vi "test Set Version on Close.vi"(8 "error in (no error)":errorcluster, 11 "TestCase in":refnum<class "Configuration Tests.lvclass">) -> (0 "error out":errorcluster, 3 "TestCase out":refnum<class "Configuration Tests.lvclass">)   [LabVIEW 2017, in "Configuration Tests.lvclass"]
uses:
  Configuration Tests.lvclass
  Typedefs/DSF Version Info.ctl
  <vilib>/addons/_JKI Toolkits/VI Tester/TestCase.llb/TestCase.lvclass
  Classes/Configuration/Configuration Session.lvclass
  DSF Core.lvlib
  C:/Program Files (x86)/National Instruments/LabVIEW 2017/vi.lib/addons/_JKI Toolkits/VI Tester/TestCase.llb/TestCase.lvclass
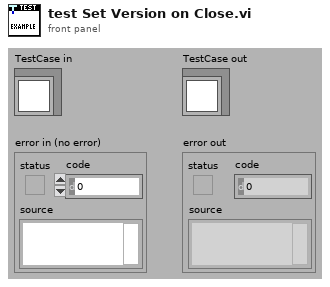
[diagram p1: front panel]
types:
  T1 = typedef "DSF Core.lvlib/DSF Version Info.ctl" = cluster{"major":u32, "minor":u32, "fix":u32, "build":string}
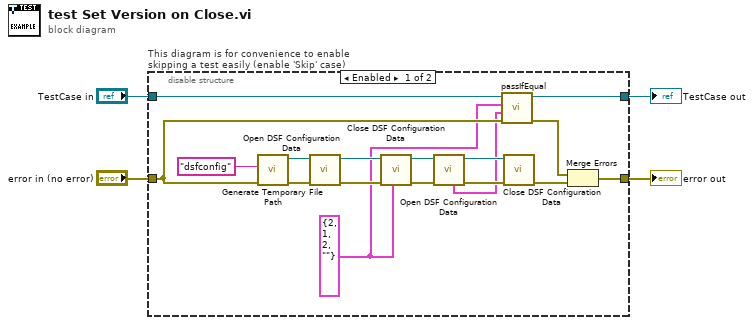
[diagram p0: block diagram]
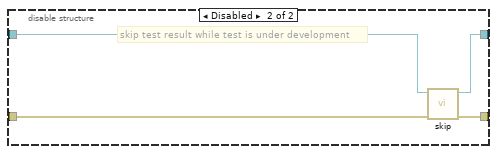
[diagram p2: hidden frame]
diagram:
  n1 = disable-structure "This diagram is for convenience to enable skipping a test easily (enable 'Skip' case)" shown="Enabled" {
    disable-tunnel: "TestCase in" -> [w18 w25]
    disable-tunnel: [w5 w23] -> w1
    disable-tunnel: [w16 w24] -> w3
    disable-tunnel: "error in (no error)" -> [w17 w22]
    frame Enabled {
      w7 = T1 {"major"=2, "minor"=1, "fix"=2, "build"=""} ("version (no change)")
      n2 = call <vilib>:"Generate Temporary File Path.vi"("error in (no error)"=w17, "Temporary File Extension (tmp)"="dsfconfig") -> ("error out"=w20:errorcluster, "Unique Temporary File Path"=w21:path)  [unwired: 8 in]
      n3 = call "Open DSF Configuration Data.vi"("error in (no error)"=w20, "dsf configuration file path"=w21) -> ("error out"=w15:errorcluster, "Configuration Session"=w13:refnum<class "Configuration Session.lvclass">)  [unwired: 5 in, 3 out]
      n4 = call "Close DSF Configuration Data.vi"("version (no change)"=w7, "error in (no error)"=w15, "Configuration Session"=w13) -> ("error out"=w14:errorcluster, "file path"=w12:path)  [unwired: 7 in]
      n5 = call "Open DSF Configuration Data.vi"("error in (no error)"=w14, "dsf configuration file path"=w12) -> ("error out"=w10:errorcluster, "Configuration Session"=w11:refnum<class "Configuration Session.lvclass">, "version"=w8:T1)  [unwired: 5 in, 2 out]
      n6 = call-dynamic "passIfEqual.vi"("error in (no error)"=w17, "y"=w8, "x"=w7, "TestCase in"=w18) -> ("error out"=w6:errorcluster, "TestCase out"=w5:refnum<class "Configuration Tests.lvclass">)  [unwired: 6 in]
      n7 = call "Close DSF Configuration Data.vi"("error in (no error)"=w10, "Configuration Session"=w11) -> ("error out"=w9:errorcluster)  [unwired: 8 in, 1 out]
      n8 = Merge Errors(w6, w9) -> (w16:errorcluster)
    }
    frame Disabled {
      # "skip test result while test is under development"
      n9 = call <vilib>:"skip.vi"("error in (no error)"=w22, "TestCase in"=w25) -> ("error out"=w24:errorcluster, "TestCase out"=w23:refnum<class "Configuration Tests.lvclass">)  [unwired: 8 in]
    }
  }
  "error out" <- w3
  "TestCase out" <- w1
